vi "Write Output_Enable.vi"(8 "error in":errorcluster, 10 "Output_Enable":bool, 11 "69X_79X in":refnum<class "6972A.lvclass">) -> (0 "error out":errorcluster, 3 "69X_79X out":refnum<class "6972A.lvclass">)   [LabVIEW 2019, in "6972A.lvlib" / "6972A.lvclass"]
uses:
  Library/6972A.lvclass
  builds/Instruments/PowerSupply.lvlibp/Library/PowerSupply.lvclass
  builds/Engine/Engine.lvlibp/Project/Engine.lvclass
  C:/Users/Public/Documents/Development/builds/Engine/Engine.lvlibp/Project/Engine.lvclass
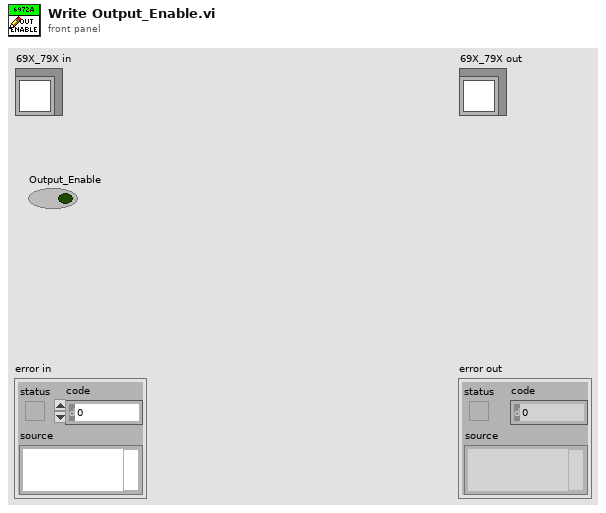
[diagram p1: front panel]
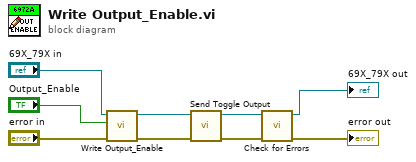
[diagram p0: block diagram]
diagram:
  n1 = call-parent "Write Output_Enable.vi"("error in"="error in", "Output_Enable"="Output_Enable", "PowerSupply in"="69X_79X in") -> ("error out"=w5:errorcluster, "PowerSupply out"=w6:refnum<class "6972A.lvclass">)  [unwired: 7 in]
  n2 = call "Send Toggle Output.vi"("error in"=w5, "69X_79X in"=w6) -> ("error out"=w3:errorcluster, "69X_79X out"=w4:refnum<class "6972A.lvclass">)  [unwired: 8 in]
  n3 = call "Check for Errors.vi"("error in"=w3, "Engine in"=w4) -> ("error out"=→"error out":errorcluster, "Engine out"=→"69X_79X out":refnum<class "6972A.lvclass">)  [unwired: 8 in]
